vi "trapwithimagePCIstandalone.vi"(3 "PulseBlaster Error In":errorcluster, 6 "Input Array 2":T1(array[cluster])=[{"Data Field"=0, "Delay"=0.01, "OP code"=0, "Output Bits"=[TRUE, FALSE, TRUE, FALSE, TRUE, FALSE, TRUE, FALSE, TRUE, FALSE, TRUE, FALSE, TRUE, FALSE, TRUE, FALSE, TRUE, FALSE, TRUE, FALSE, TRUE, FALSE, TRUE, FALSE], "String"=""}, {"Data Field"=0, "Delay"=0.01, "OP code"=0, "Output Bits"=[FALSE, TRUE, FALSE, TRUE, FALSE, TRUE, FALSE, TRUE, FALSE, TRUE, FALSE, TRUE, FALSE, TRUE, FALSE, TRUE, FALSE, TRUE, FALSE, TRUE, FALSE, TRUE, FALSE, TRUE], "String"=""}, {"Data Field"=0, "Delay"=0.01, "OP code"=0, "Output Bits"=[TRUE, FALSE, TRUE, FALSE, TRUE, FALSE, TRUE, FALSE, TRUE, FALSE, TRUE, FALSE, TRUE, FALSE, TRUE, FALSE, TRUE, FALSE, TRUE, FALSE, TRUE, FALSE, TRUE, FALSE], "String"=""}, {"Data Field"=0, "Delay"=0.01, "OP code"=0, "Output Bits"=[FALSE, TRUE, FALSE, TRUE, FALSE, TRUE, FALSE, TRUE, FALSE, TRUE, FALSE, TRUE, FALSE, TRUE, FALSE, TRUE, FALSE, TRUE, FALSE, TRUE, FALSE, TRUE, FALSE, TRUE], "String"=""}, {"Data Field"=0, "Delay"=0.01, "OP code"=0, "Output Bits"=[TRUE, FALSE, TRUE, FALSE, TRUE, FALSE, TRUE, FALSE, TRUE, FALSE, TRUE, FALSE, TRUE, FALSE, TRUE, FALSE, TRUE, FALSE, TRUE, FALSE, TRUE, FALSE, TRUE, FALSE], "String"=""}, {"Data Field"=0, "Delay"=0.01, "OP code"=6, "Output Bits"=[FALSE, TRUE, FALSE, TRUE, FALSE, TRUE, FALSE, TRUE, FALSE, TRUE, FALSE, TRUE, FALSE, TRUE, FALSE, TRUE, FALSE, TRUE, FALSE, TRUE, FALSE, TRUE, FALSE, TRUE], "String"="\"Go To\" sends you to col. 0"}, {"Data Field"=0, "Delay"=0.01, "OP code"=0, "Output Bits"=[FALSE, FALSE, FALSE, FALSE, FALSE, FALSE, FALSE, FALSE, FALSE, FALSE, FALSE, FALSE, FALSE, FALSE, FALSE, FALSE, FALSE, FALSE, FALSE, FALSE, FALSE, FALSE, FALSE, FALSE], "String"=""}, {"Data Field"=0, "Delay"=0.01, "OP code"=0, "Output Bits"=[FALSE, FALSE, FALSE, FALSE, FALSE, FALSE, FALSE, FALSE, FALSE, FALSE, FALSE, FALSE, FALSE, FALSE, FALSE, FALSE, FALSE, FALSE, FALSE, FALSE, FALSE, FALSE, FALSE, FALSE], "String"=""}, {"Data Field"=0, "Delay"=0.01, "OP code"=0, "Output Bits"=[FALSE, FALSE, FALSE, FALSE, FALSE, FALSE, FALSE, FALSE, FALSE, FALSE, FALSE, FALSE, FALSE, FALSE, FALSE, FALSE, FALSE, FALSE, FALSE, FALSE, FALSE, FALSE, FALSE, FALSE, FALSE], "String"=""}, {"Data Field"=0, "Delay"=0.01, "OP code"=0, "Output Bits"=[FALSE, FALSE, FALSE, FALSE, FALSE, FALSE, FALSE], "String"=""}, {"Data Field"=0, "Delay"=0.01, "OP code"=0, "Output Bits"=[FALSE, FALSE, FALSE, FALSE, FALSE, FALSE], "String"=""}, {"Data Field"=0, "Delay"=0.01, "OP code"=0, "Output Bits"=[FALSE, FALSE, FALSE, FALSE, FALSE, FALSE], "String"=""}, {"Data Field"=0, "Delay"=0.01, "OP code"=0, "Output Bits"=[FALSE, FALSE, FALSE, FALSE, FALSE, FALSE], "String"=""}, {"Data Field"=0, "Delay"=0.01, "OP code"=0, "Output Bits"=[FALSE, FALSE, FALSE, FALSE, FALSE, FALSE], "String"=""}, {"Data Field"=0, "Delay"=0.01, "OP code"=0, "Output Bits"=[FALSE], "String"=""}, {"Data Field"=0, "Delay"=0.01, "OP code"=0, "Output Bits"=[FALSE, FALSE, FALSE, FALSE, FALSE, FALSE, FALSE, FALSE, FALSE, FALSE, FALSE, FALSE, FALSE, FALSE, FALSE, FALSE, FALSE, FALSE, FALSE, FALSE, FALSE, FALSE, FALSE, FALSE, FALSE], "String"=""}, {"Data Field"=0, "Delay"=0.01, "OP code"=0, "Output Bits"=[], "String"=""}, {"Data Field"=0, "Delay"=0.01, "OP code"=0, "Output Bits"=[], "String"=""}, {"Data Field"=0, "Delay"=0.01, "OP code"=0, "Output Bits"=[], "String"=""}, {"Data Field"=0, "Delay"=0.01, "OP code"=6, "Output Bits"=[FALSE, FALSE, FALSE, FALSE, FALSE, FALSE, FALSE, FALSE, FALSE], "String"=""}] {"OP code" items=["Continue", "Stop", "Loop", "End Loop", "Jump", "Return", "Go To", "Long Delay", "Wait"]; "Delay" format="%.3p"}) -> (0 "error out":errorcluster)   [LabVIEW 2013]
doc: "This VI allows one to program a PulseBlaster board's channels without having to deal with the \"very long instruction word\" (VLIW) commands directly. One ought to consult the reference material in the \"Programming the PulseBlaster: Instruction Set Architecture\" section of the manual for more information.\n\nThe default settings should output HI-LO-HI in 10 ms intervals on even-numbered channels and LO-HI-LO on odd-numbered channels. The default settings use the first 6 columns of input; note that the first 5 columns use the \"Continue\" command while the sixth column specifies \"Go To\" column zero to create the loop.\n\nThis VI was originally created at NIST circa 2001. Since then, the Killian Lab at Rice University has adapted it for use in their lab. Most recently, it has been converted for use on PCI versions of Spincore's PulseBlaster series of boards in the Killian Lab. Support is not guaranteed, but questions may be directed to Pascal Mickelson at mickelsp@rice.edu."
panel:
  in  "Listbox":i32(listbox)=13
  in  "file path (dialog if empty)":path=path "c:/data/junk"
  out "Written Instruction Array":T2(array[cluster])=[{"Output Bits"=5592405, "Data Field"=0, 0, 999997}, {"Output Bits"=11184810, "Data Field"=0, 0, 999997}, {"Output Bits"=5592405, "Data Field"=0, 0, 999997}, {"Output Bits"=11184810, "Data Field"=0, 0, 999997}, {"Output Bits"=5592405, "Data Field"=0, 0, 999997}, {"Output Bits"=11184810, "Data Field"=0, 6, 999997}, {"Output Bits"=0, "Data Field"=0, 0, 999997}, {"Output Bits"=0, "Data Field"=0, 0, 999997}, {"Output Bits"=0, "Data Field"=0, 0, 999997}, {"Output Bits"=0, "Data Field"=0, 0, 999997}, {"Output Bits"=0, "Data Field"=0, 0, 999997}, {"Output Bits"=0, "Data Field"=0, 0, 999997}, {"Output Bits"=0, "Data Field"=0, 0, 999997}, {"Output Bits"=0, "Data Field"=0, 0, 999997}, {"Output Bits"=0, "Data Field"=0, 0, 999997}, {"Output Bits"=0, "Data Field"=0, 0, 999997}, {"Output Bits"=0, "Data Field"=0, 0, 999997}, {"Output Bits"=0, "Data Field"=0, 0, 999997}, {"Output Bits"=0, "Data Field"=0, 0, 999997}, {"Output Bits"=0, "Data Field"=0, 6, 999997}]
  out "Actual Delays":dbl[](array[numeric])=[0.01, 0.01, 0.01, 0.01, 0.01, 0.01, 0.01, 0.01, 0.01, 0.01, 0.01, 0.01, 0.01, 0.01, 0.01, 0.01, 0.01, 0.01, 0.01, 0.01] format="%.9f"
  # "1st column is 0, 1st Boolean is 1 (24 Booleans allowed). 20 words shown (can be expanded). \nTime: 1= 1sec., 1m=1millisec, 1u= 1 microsec. 10n=10 nanosec.; time will be rounded to 10ns steps\n         (and 30 ns delay is added)"
  # "All bits have to be set low at the last statement\nbefore the `stop' /'wait' command."
  # "Data on file:\nOutput pattern | Data Field | Op Code | Delay"
  # "Delay (cycles)"
  # "Op code"
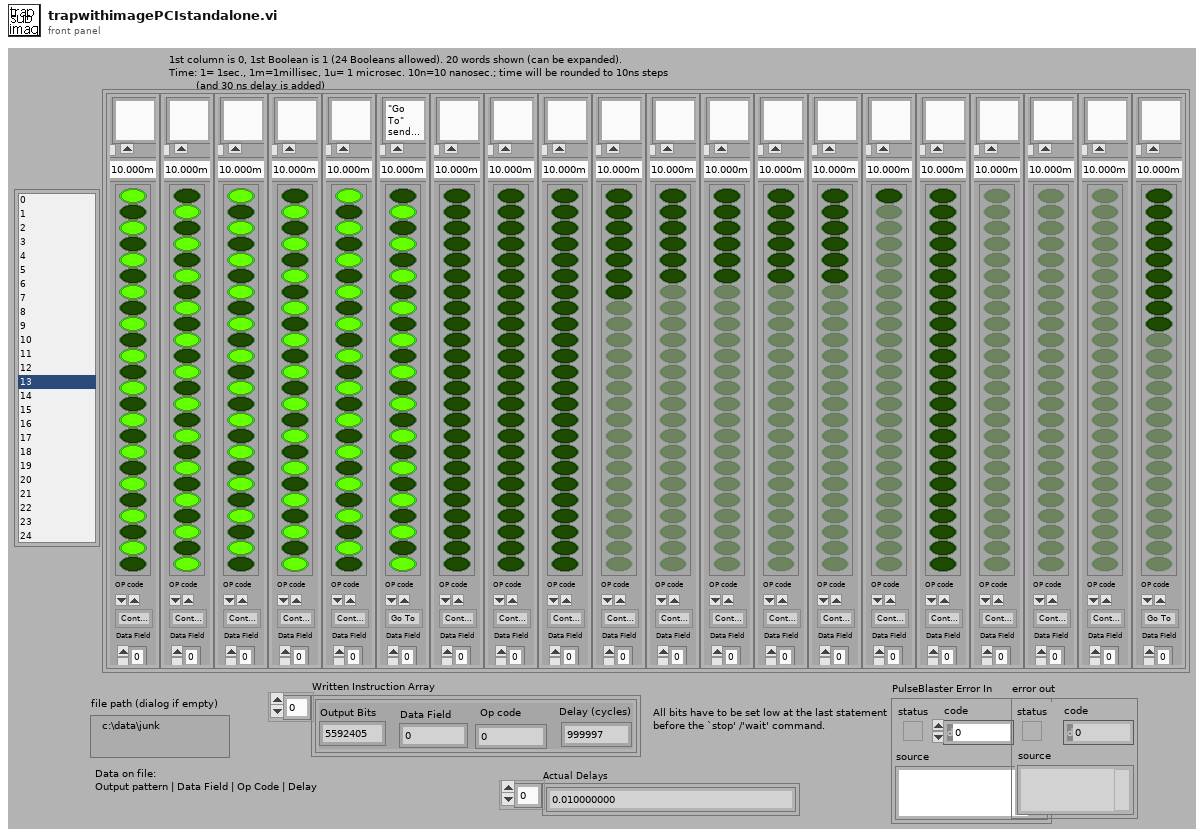
[diagram p1: front panel]
types:
  T1 = cluster{"Data Field":u32, "Delay":dbl, "OP code":u8, "Output Bits":bool[], "String":string}[]
  T2 = cluster{"Output Bits":u32, "Data Field":u32, u32, u32}[]
  T3 = cluster{"Output Bits":u32, "Data Field":u32, "Delay Count":u32, "OP Code":u8}[]
  T4 = cluster{"Output Bits":u32, "Data Field":u32, "OP Code":u8, "Delay Count":u32}[]
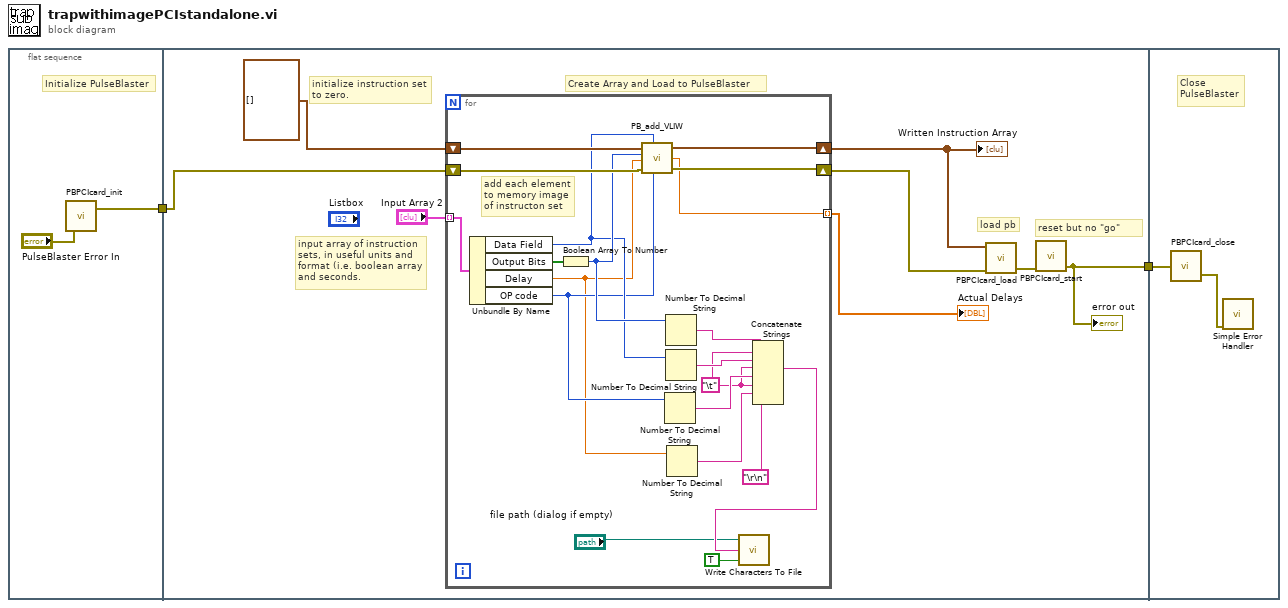
[diagram p0: block diagram]
diagram:
  n1 = flat-sequence {
    tunnel: [w3] -> w1
    tunnel: [w9] -> w2
    tunnel: w1 -> [w5]
    tunnel: w2 -> [w34]
    frame #0 {
      # "Initialize PulseBlaster"
      n2 = call "PBPCIcard_init.vi"("error in"="PulseBlaster Error In") -> ("error out"=w3:errorcluster)  [unwired: 1 out]
    }
    frame #1 {
      # "Create Array and Load to PulseBlaster"
      # "input array of instruction\nsets, in useful units and\nformat (i.e. boolean array\nand seconds."
      # "initialize instruction set\nto zero."
      # "reset but no \"go\""
      # "load pb"
      n3 = for {
        shift-right: [w32] -> w7
        shift-left: T3 [] ("VLIW Array In") -> [w31]
        shift-right: [w30] -> w12
        shift-left: w5 -> [w29]
        tunnel: [w28] -> w10 mode=indexing
        tunnel: "Input Array 2" -> [w26] mode=indexing
        w21 = "\t"
        # "add each element\nto memory image\nof instructon set"
        n4 = Unbundle By Name(w26) -> ("Data Field"=w15:u32, "Output Bits"=w27:bool[], "Delay"=w13:dbl, "OP code"=w14:u8)
        n5 = Boolean Array To Number(Boolean array=w27) -> (number=w16:u32)
        n6 = call "PB_add_VLIW.vi"("VLIW Array In"=w31, "Data Field"=w15, "Digital Bits"=w16, "Delay"=w13, "OP code"=w14, "error in (no error)"=w29) -> ("VLIW Array Out"=w32:T4, "Actual Delay"=w28:dbl, "error out"=w30:errorcluster)
        n7 = Number To Decimal String(number=w14) -> (decimal integer string=w23:string)  [unwired: 1 in]
        n8 = Number To Decimal String(number=w16) -> (decimal integer string=w25:string)  [unwired: 1 in]
        n9 = Number To Decimal String(number=w15) -> (decimal integer string=w24:string)  [unwired: 1 in]
        n10 = Number To Decimal String(number=w13) -> (decimal integer string=w22:string)  [unwired: 1 in]
        n11 = Concatenate Strings(w25, w21, w24, w21, w23, w21, w22, "\r\n") -> (w19:string)
        n12 = call <vilib>:"Write Characters To File.vi"("append to file? (new file:F)"=TRUE, "character string"=w19, "file path (dialog if empty)"="file path (dialog if empty)") -> ()  [unwired: 2 in, 1 out]
      }
      "Actual Delays" <- w10
      "Written Instruction Array" <- w7
      n13 = call "PBPCIcard_load.vi"("PulseBlaster\nVLIW Array"=w7, "error in (no error)"=w12) -> ("error out"=w11:errorcluster)  [unwired: 5 in]
      n14 = call "PBPCIcard_start.vi"("error in (no error)"=w11) -> ("error out"=w9:errorcluster)  [unwired: 6 in]
      "error out" <- w9
    }
    frame #2 {
      # "Close\nPulseBlaster"
      n15 = call "PBPCIcard_close.vi"("error in"=w34) -> ("error out"=w33:errorcluster)  [unwired: 1 out]
      n16 = call <vilib>:"Simple Error Handler.vi"("error in (no error)"=w33) -> ()  [unwired: 4 in, 5 out]
    }
  }
